vi "Export_Data_From_TXT_With_Menu_v1.0.vi"() -> ()   [LabVIEW 2018]
panel:
  out "array":dbl[][](array[numeric])
  in  "Open":bool
  in  "Выбор файла":path
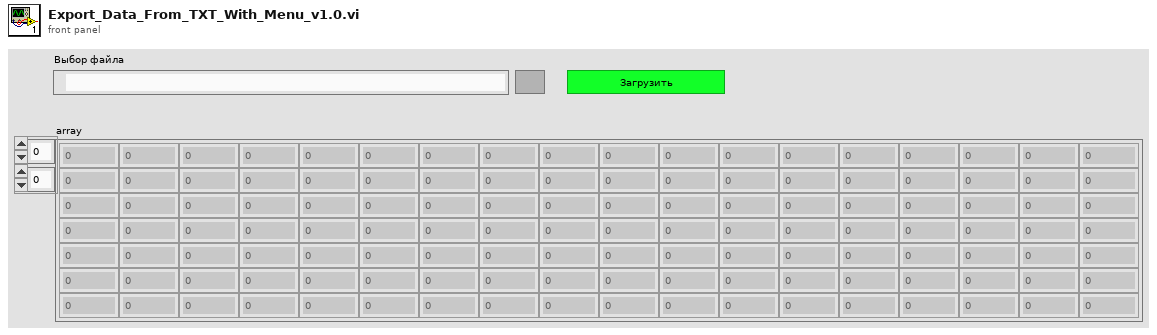
[diagram p1: front panel]
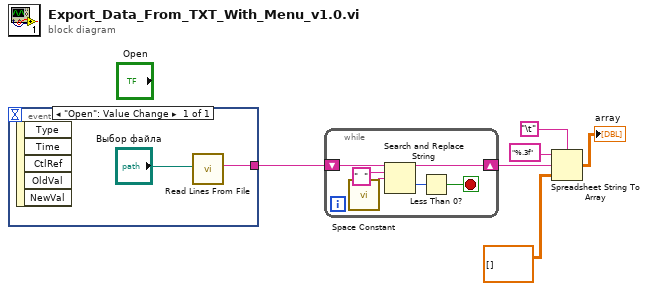
[diagram p0: block diagram]
diagram:
  n1 = event shown="[0] \"Open\": Value Change" {
    selector: _ -> [_]
    dyn-events: _ -> [_]
    timeout: _ -> [_]
    tunnel: [w8] -> w1
    event "Open": Value Change {
      n2 = event-data() -> ()  [unwired: 1 in, 5 out]
      n3 = call <vilib>:"Read Lines From File.vi"("file path (dialog if empty)"="Выбор файла") -> ("line string"=w8:string)  [unwired: 1 in, 7 out]
    }
  }
  n4 = while {
    shift-right: [w11] -> w4
    shift-left: w1 -> [w14]
    stop <- w9 stop-if-true
    n5 = call <vilib>:"Space Constant.vi"() -> ("String"=w12:string)
    n6 = Search and Replace String(input string=w14, search string="  ", replace string=w12) -> (result string=w11:string, offset past replacement=w10:i32)  [unwired: 1 in, 6 out]
    n7 = Less Than 0?(x=w10) -> (x < 0?=w9:bool)
  }
  n8 = Spreadsheet String To Array(delimiter (Tab)="\t", format string="%.3f" ("format (%.3f)"), spreadsheet string=w4, array type (2D Dbl)=dbl[][] [] ("type (empty)")) -> (array=→"array":dbl[][])
